vi "Measure Output.vi"(8 "error in":errorcluster, 11 "6700C in":refnum<class "6700C.lvclass">) -> (0 "error out":errorcluster, 1 "Current":dbl[](array[numeric]), 2 "Voltage":dbl[](array[numeric]), 3 "6700C out":refnum<class "6700C.lvclass">)   [LabVIEW 2019, in "6700C.lvlib" / "6700C.lvclass"]
uses:
  Library/6700C.lvclass
  C:/Users/Public/Documents/Development/builds/Instruments/PowerSupply.lvlibp/Library/PowerSupply.lvclass
  builds/Instruments/PowerSupply.lvlibp/Private/Accessors/Read Number of Channels.vi
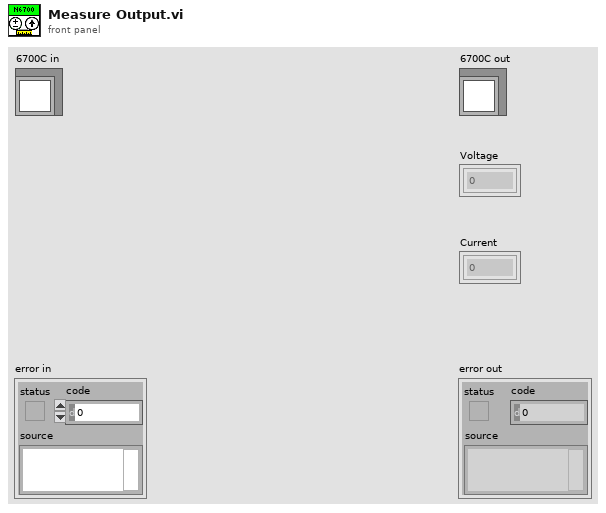
[diagram p1: front panel]
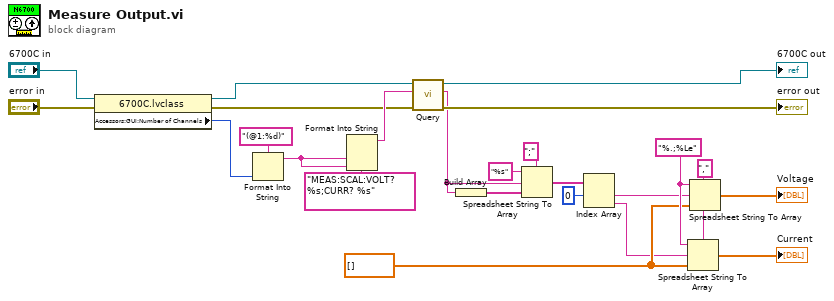
[diagram p0: block diagram]
diagram:
  w9 = "," ("delimiter (Tab)")
  w7 = dbl[] []
  w8 = "%.;%Le"
  n1 = property class="6700C.lvclass"(reference="6700C in", error in="error in") -> (reference out=w18:refnum<class "6700C.lvclass">, error out=w15:errorcluster, "Accessors:GUI:Number of Channels"=w20:i32)
  n2 = Format Into String(format string="(@1:%d)", w20) -> (resulting string=w24:string)  [unwired: 2 in, 1 out]
  n3 = Format Into String(format string="MEAS:SCAL:VOLT? %s;CURR? %s", w24, w24) -> (resulting string=w17:string)  [unwired: 2 in, 1 out]
  n4 = call "Query.vi"("error in"=w15, "Write in"=w17, "6700C in"=w18) -> ("error out"=→"error out":errorcluster, "Read out"=w10:string, "6700C out"=→"6700C out":refnum<class "6700C.lvclass">)  [unwired: 6 in]
  n5 = Build Array(w10) -> (w13:string[])
  n6 = Spreadsheet String To Array(delimiter (Tab)=";", format string="%s", spreadsheet string=w10, array type (2D Dbl)=w13) -> (array=w6:string[])
  n7 = Index Array(array=w6, index #1=0 ("index")) -> (element #1=w4:string, element #2=w3:string)  [unwired: 1 in]
  n8 = Spreadsheet String To Array(delimiter (Tab)=w9, format string=w8, spreadsheet string=w3, array type (2D Dbl)=w7) -> (array=→"Current":dbl[])
  n9 = Spreadsheet String To Array(delimiter (Tab)=w9, format string=w8, spreadsheet string=w4, array type (2D Dbl)=w7) -> (array=→"Voltage":dbl[])
